vi "nocsec.vi"() -> ()   [LabVIEW 2011]
uses:
  <vilib>/Utility/config.llb/Read Key (String).vi
  <vilib>/Utility/config.llb/NI_LVConfig.lvlib
panel:
  out "element":string
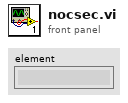
[diagram p1: front panel]
types:
  T1 = typedef "NI_LVConfig.lvlib/Config Data RefNum.ctl" = refnum<k1>
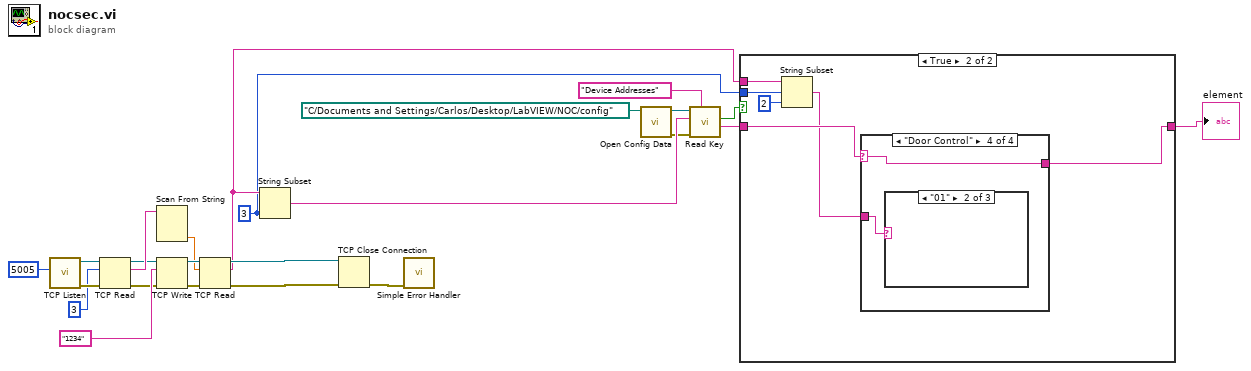
[diagram p0: block diagram]
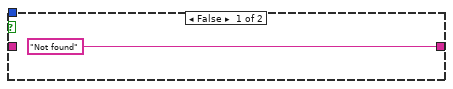
[diagram p2: hidden frame]
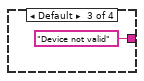
[diagram p5: hidden frame]
diagram:
  w1 = 3 ("length (rest)")
  n1 = call <vilib>:"TCP Listen.vi"("port"=u16 5005) -> ("error out"=w23:errorcluster, "connection ID"=w22:refnum<k5>)  [unwired: 6 in, 3 out]
  n2 = TCP Read(connection ID=w22, bytes to read=3, error in (no error)=w23) -> (connection ID out=w17:refnum<k5>, data out=w18:string, error out=w16:errorcluster)  [unwired: 2 in]
  n3 = Scan From String(input string=w18) -> (output 1=w13:dbl)  [unwired: 4 in, 3 out]
  n4 = TCP Write(connection ID=w17, data in="1234" ("response"), error in (no error)=w16) -> (connection ID out=w15:refnum<k5>, error out=w14:errorcluster)  [unwired: 1 in, 1 out]
  n5 = TCP Read(connection ID=w15, bytes to read=w13, error in (no error)=w14) -> (connection ID out=w11:refnum<k5>, data out=w2:string, error out=w12:errorcluster)  [unwired: 2 in]
  n6 = String Subset(string=w2, length (rest)=w1) -> (substring=w6:string)  [unwired: 1 in]
  n7 = TCP Close Connection(connection ID=w11, error in (no error)=w12) -> (error out=w24:errorcluster)  [unwired: 1 in, 1 out]
  n8 = call <vilib>:"Simple Error Handler.vi"("error in (no error)"=w24) -> ()  [unwired: 4 in, 5 out]
  n9 = call <vilib>:"Open Config Data.vi"("configuration file path"=path "C:/Documents and Settings/Carlos/Desktop/LabVIEW/NOC/config") -> ("error out"=w5:errorcluster, "refnum"=w7:T1)  [unwired: 8 in, 1 out]
  n10 = call-poly <vilib>:"Read Key.vi"("section"="Device Addresses", "error in (no error)"=w5, "key"=w6, "refnum"=w7) -> ("value"=w9:string, "found?"=w4:bool)  [unwired: 4 in, 2 out]
  n11 = case shown="True" w4 {
    tunnel: w9 -> [_ w28]
    tunnel: ["Not found" ("value") w27] -> w3
    tunnel: w2 -> [_ w30]
    tunnel: w1 -> [_ w29]
    frame False {
    }
    frame True {
      n12 = String Subset(string=w30, offset (0)=w29, length (rest)=2 ("length (rest)")) -> (substring=w26:string)
      n13 = case shown="\"Door Control\"" w28 {
        selector: w28 -> [w32 w33 _ w36]
        tunnel: [w32 w33 "Device not valid" w36] -> w27
        tunnel: w26 -> [_ _ _ w35]
        frame "Lights" {
        }
        frame "Portable 1" {
        }
        frame Default {
        }
        frame "Door Control" {
          n14 = case shown="\"01\"" w35 {
            frame Default {
            }
            frame "01" {
            }
            frame "00" {
            }
          }
        }
      }
    }
  }
  "element" <- w3
